vi "SPIN2_Hybrid_ODFT_Meas.vi"(0 "Semiconductor Module Context":T1, 1 "PI_1_Meas":dbl format="%#_6p", 2 "script name":string="ODFTwHV0", 5 "Pins":string[](array[string])=["HV"], 7 "Publishable IDs":string[](array[string])=["IDD_LowPower", "IDD_DVC_Cmin", "IDD_DVC_Cmax"], 9 "Delay Time (s)":dbl=0.001 format="%#_13p", 12 "Ext_HV":dbl=41.25 format="%#_6p") -> (15 "error out":errorcluster)   [LabVIEW 2013]
uses:
  <vilib>/NI_TestStand_SemiconductorModule/NI_TestStand_Semiconductor_Module.lvlibp/PinMap/General/SemiconductorModuleContext.ctl
  <instrlib>/niHSDIO/niHSDIO.llb/niHSDIO_ctl Trigger Script - trigID Values (Ring).ctl
  <vilib>/NI_TestStand_SemiconductorModule/NI_TestStand_Semiconductor_Module.lvlibp/PinMap/DC Power/PinsToNIDCPowerSessions.vi
  <vilib>/NI_TestStand_SemiconductorModule/NI_TestStand_Semiconductor_Module.lvlibp/PinMap/Deprecated/PublishDataDoubleMultiplePinsMultipleInstruments.vi
  <vilib>/NI_TestStand_SemiconductorModule/NI_TestStand_Semiconductor_Module.lvlibp/PinMap/Deprecated/PublishDataDoubleMultiplePinsSingleInstrument.vi
  <vilib>/NI_TestStand_SemiconductorModule/NI_TestStand_Semiconductor_Module.lvlibp
panel:
  out "iPI_Calc":dbl[](array[numeric])
  out "current measurements":dbl[][](array[numeric])
  out "Delta_iHV_Measurements":dbl[][](array[numeric])
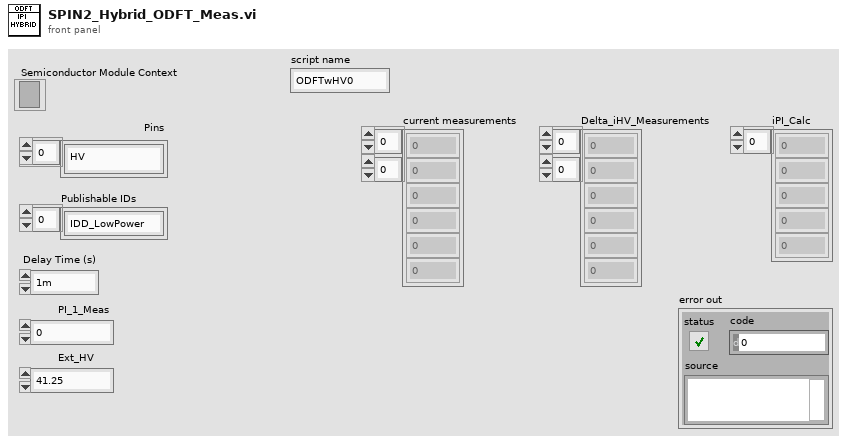
[diagram p1: front panel]
types:
  T1 = typedef "NI_TestStand_Semiconductor_Module.lvlibp/SemiconductorModuleContext.ctl" = refnum<k7>
  T2 = typedef "niHSDIO_ctl Trigger Script - trigID Values (Ring).ctl" = string
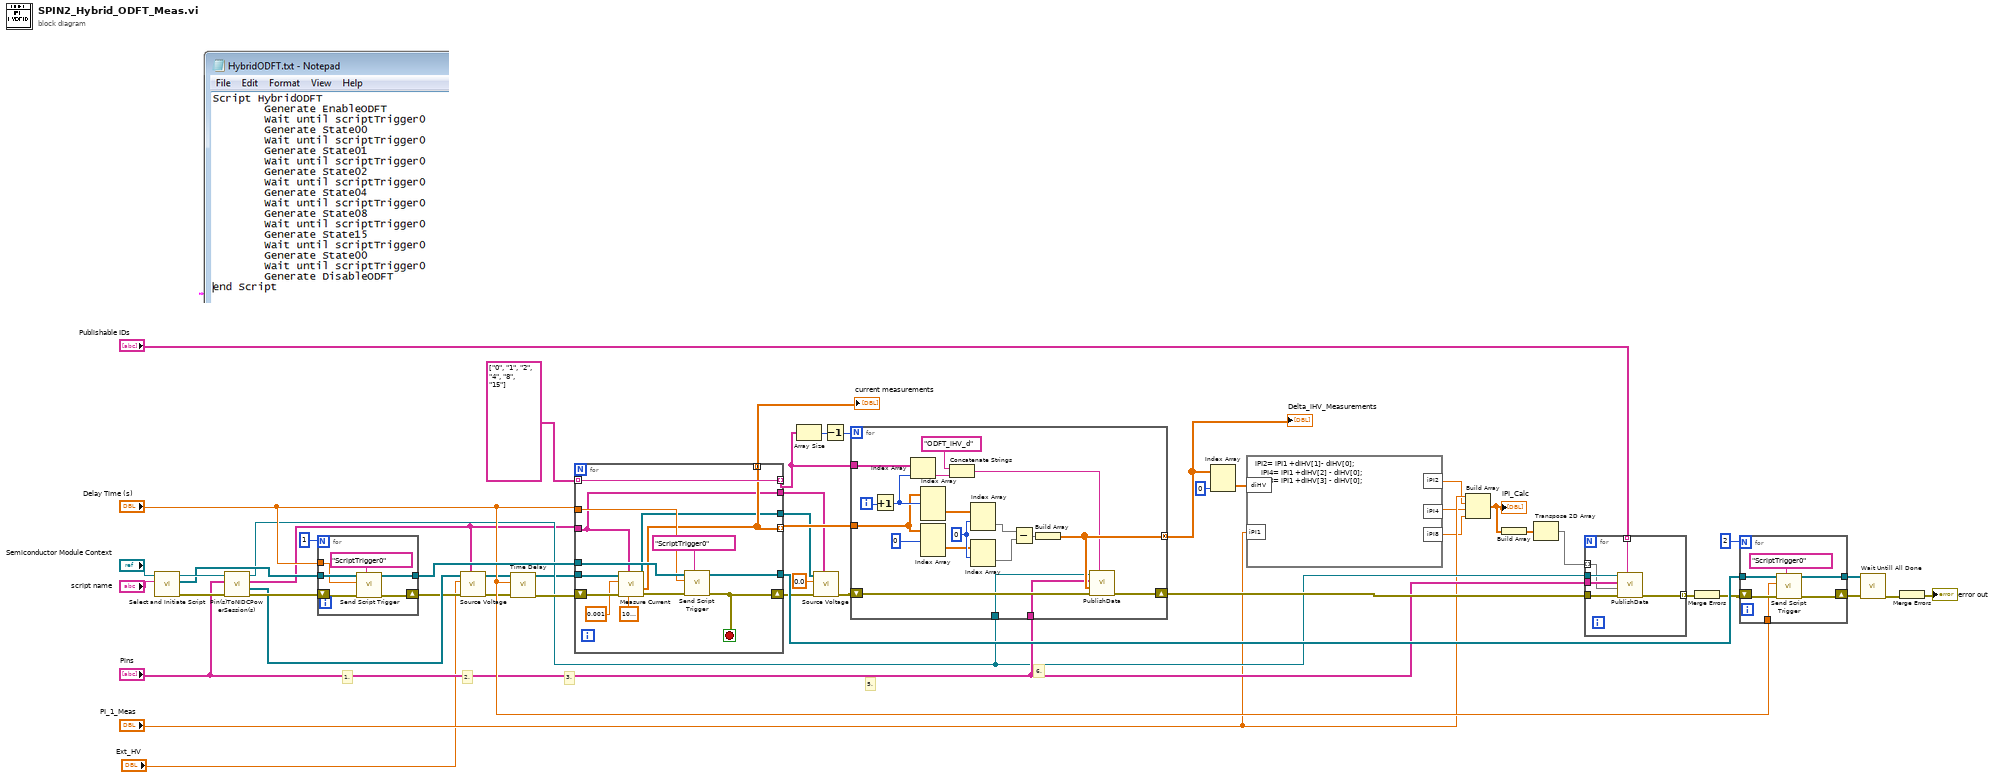
[diagram p0: block diagram]
diagram:
  # "3."
  # "6."
  # "5."
  # "2."
  # "1."
  n1 = call "Select and Initiate Script.vi"("script name"="script name", "Semiconductor Module Context"="Semiconductor Module Context") -> ("error out"=w38:errorcluster, "HSDIO GEN Sessions Out"=w39:refnum<k15>[], "Semiconductor Module Context Out"=w40:T1)  [unwired: 7 in]
  n2 = call-poly <vilib>:"Pin(s)ToNIDCPowerSession(s).vi"("error in (no error)"=w38, "Pins"="Pins", "Semiconductor Module Context"=w40) -> ("error out"=w48:errorcluster, "Instrument Sessions"=w11:refnum<k15>[], "Channel Lists"=w7:string[], "Semiconductor Module Context Out"=w16:T1)  [unwired: 4 in, 1 out]
  n3 = for {
    N: 1 -> [_]
    shift-right: [w53] -> w9
    shift-left: w48 -> [w54]
    tunnel: w39 -> [w52]
    tunnel: [w51] -> w36
    tunnel: "Delay Time (s)" -> [w50]
    n4 = call "Send Script Trigger.vi"("trigger id (script trigger 0)"=T2 "ScriptTrigger0", "error in (no error)"=w54, "Delay Time (s)"=w50, "HSDIO Sessions In"=w52) -> ("error out"=w53:errorcluster, "HSDIO Sessions Out"=w51:refnum<k15>[])  [unwired: 6 in]
  }
  n5 = call "Source Voltage.vi"("Channel Lists"=w7, "error in (no error)"=w9, "voltage level"="Ext_HV", "Instrument Sessions In"=w11) -> ("error out"=w8:errorcluster, "Instrument Sessions Out"=w10:refnum<k15>[])  [unwired: 4 in, 2 out]
  n6 = call "Time Delay"("error in (no error)"=w8, "Delay Time (s)"="Delay Time (s)") -> ("error out"=w34:errorcluster)  [unwired: 9 in]
  n7 = for {
    tunnel: string[] ["0", "1", "2", "4", "8", "15"] -> [w69] mode=indexing
    tunnel: w10 -> [w64]
    shift-right: [w66] -> w5
    shift-left: w34 -> [w65]
    tunnel: [w69] -> w45 mode=indexing
    tunnel: w36 -> [w67]
    tunnel: w7 -> [w56]
    tunnel: [w59] -> w35 mode=indexing
    tunnel: [w61] -> w33
    tunnel: "Delay Time (s)" -> [w60]
    tunnel: [w59] -> w28 mode=concatenating
    tunnel: [w57] -> w2
    tunnel: [w56] -> w1
    stop <- w66 stop-if-true
    n8 = call "Measure Current.vi"("Result Multiplier"=1000000.0, "Channel Lists"=w56, "error in (no error)"=w65, "Delay Time (s)"=0.001, "DCPower Sessions In"=w64) -> ("error out"=w58:errorcluster, "current measurements"=w59:dbl[][], "DCPower Sessions Out"=w57:refnum<k15>[])  [unwired: 4 in]
    n9 = call "Send Script Trigger.vi"("trigger id (script trigger 0)"=T2 "ScriptTrigger0", "error in (no error)"=w58, "Delay Time (s)"=w60, "HSDIO Sessions In"=w67) -> ("error out"=w66:errorcluster, "HSDIO Sessions Out"=w61:refnum<k15>[])  [unwired: 6 in]
  }
  "current measurements" <- w28
  n10 = Array Size(array=w45) -> (size(s)=w44:i32)
  n11 = call "Source Voltage.vi"("Channel Lists"=w1, "error in (no error)"=w5, "voltage level"=0.0, "Instrument Sessions In"=w2) -> ("error out"=w4:errorcluster)  [unwired: 4 in, 3 out]
  n12 = Decrement(x=w44) -> (x-1=w43:i32)
  n13 = for {
    N: w43 -> [_]
    tunnel: w45 -> [w86]
    shift-right: [w75] -> w24
    shift-left: w4 -> [w74]
    tunnel: w35 -> [w81]
    tunnel: [w73] -> w25 mode=concatenating
    tunnel: "Pins" -> [w71]
    tunnel: w16 -> [w70]
    i -> [w87]
    w82 = 0 ("index (page)")
    n14 = Increment(x=w87) -> (x+1=w83:i32)
    n15 = Index Array(array=w86, index=w83) -> (element=w85:string)
    n16 = Index Array(array=w81, index (dim 0)=w83) -> (element=w80:dbl[][])  [unwired: 2 in]
    n17 = Index Array(array=w81, index (dim 0)=0 ("index (page)")) -> (element=w79:dbl[][])  [unwired: 2 in]
    n18 = Concatenate Strings("ODFT_iHV_d", w85) -> (w72:string)
    n19 = Index Array(array=w80, index (row)=w82) -> (element=w77:dbl[])  [unwired: 1 in]
    n20 = Index Array(array=w79, index (row)=w82) -> (element=w78:dbl[])  [unwired: 1 in]
    n21 = Subtract(x=w77, y=w78) -> (x-y=w76:dbl[])
    n22 = Build Array(w76) -> (w73:dbl[][])
    n23 = call-poly <vilib>:"PublishData.vi"("Measurement Id"=w72, "error in (no error)"=w74, "Data In"=w73, "Pins"=w71, "Semiconductor Module Context"=w70) -> ("error out"=w75:errorcluster)  [unwired: 5 in, 1 out]
  }
  "Delta_iHV_Measurements" <- w25
  n24 = Index Array(array=w25, index (col)=0 ("disabled index (col)")) -> (element=w26:dbl[])  [unwired: 1 in]
  n25 = formula code="iPI2= iPI1 +diHV[1]- diHV[0];\n   iPI4= iPI1 +diHV[2] - diHV[0];\n   iPI8= iPI1 +diHV[3] - diHV[0];"("diHV"=w26, "iPI1"="PI_1_Meas") -> ("iPI2"=w14:dbl, "iPI4"=w13:dbl, "iPI8"=w12:dbl)
  n26 = Build Array("PI_1_Meas", w14, w13, w12) -> (w20:dbl[])
  "iPI_Calc" <- w20
  n27 = Build Array(w20) -> (w19:dbl[][])
  n28 = Transpose 2D Array(2D array=w19) -> (transposed array=w18:dbl[][])
  n29 = for {
    tunnel: w24 -> [w94]
    tunnel: [w93] -> w23 mode=indexing
    tunnel: "Pins" -> [w91]
    tunnel: w16 -> [w92]
    tunnel: "Publishable IDs" -> [w90] mode=indexing
    tunnel: w18 -> [w89] mode=indexing
    n30 = call-poly <vilib>:"PublishData.vi"("Measurement Id"=w90, "error in (no error)"=w94, "Data In"=w89, "Pins"=w91, "Semiconductor Module Context"=w92) -> ("error out"=w93:errorcluster)  [unwired: 5 in, 1 out]
  }
  n31 = Merge Errors(w23) -> (w22:errorcluster)
  n32 = for {
    N: 2 -> [_]
    shift-right: [w98] -> w31
    shift-left: w22 -> [w99]
    tunnel: w33 -> [w97]
    tunnel: [w96] -> w32
    tunnel: "Delay Time (s)" -> [w95]
    n33 = call "Send Script Trigger.vi"("trigger id (script trigger 0)"=T2 "ScriptTrigger0", "error in (no error)"=w99, "Delay Time (s)"=w95, "HSDIO Sessions In"=w97) -> ("error out"=w98:errorcluster, "HSDIO Sessions Out"=w96:refnum<k15>[])  [unwired: 6 in]
  }
  n34 = call "Wait Untill All Done.vi"("error in (no error)"=w31, "HSDIO Sessions In"=w32) -> ("error out"=w37:errorcluster)  [unwired: 8 in, 1 out]
  n35 = Merge Errors(w37) -> (→"error out":errorcluster)
